vi "Valve automation test.vi"() -> ()   [LabVIEW 2016]
uses:
  <vilib>/Analysis/baseanly.llb/Mean (DBL).vi
  <vilib>/Analysis/NI_AALPro.lvlib
  <vilib>/Analysis/NI_AALBase.lvlib
  <vilib>/addons/control/pid/NI_PID_autopid.lvlib
panel:
  in  "PID gains":T1={"proportional gain (Kc)"=1.0, "integral time (Ti, min)"=0.01, "derivative time (Td, min)"=0.0} {"derivative time (Td, min)" format="%.3f"; "integral time (Ti, min)" format="%.3f"; "proportional gain (Kc)" format="%.3f"}
  out "PID gains out":T1={"proportional gain (Kc)"=1.0, "integral time (Ti, min)"=0.01, "derivative time (Td, min)"=0.0} {"derivative time (Td, min)" format="%.3f"; "integral time (Ti, min)" format="%.3f"; "proportional gain (Kc)" format="%.3f"}
  out "criterion":dbl
  out "output":dbl format="%.2f"
  out "new fill time":dbl
  out "abs error":dbl[unit]
  out "rate":dbl
  out "rel error":dbl
  in  "initial fill/vac tol":dbl
  in  "Samples to average":i32
  in  "Run":bool
  in  "Vacuum Cutoff":dbl[unit]
  in  "Fill Cutoff":dbl[unit]
  out "System Pressures":T2(graph)
  in  "Stop Button 2":bool
  in  "State":u16(ring) items=["Hold", "Vacuum", "Fill", "Vent"]
  out "Tube Inlet State":bool
  out "Mix Inlet State":bool
  out "Mix Outlet State":bool
  out "Tube Outlet State":bool
  out "Diluent State 2":bool caption="Diluent State"
  out "Vacuum State 2":bool caption="Vacuum State"
  out "Tube Pressure":dbl[unit]
  out "Manifold Pressure":dbl[unit]
  in  "Stop Button":bool
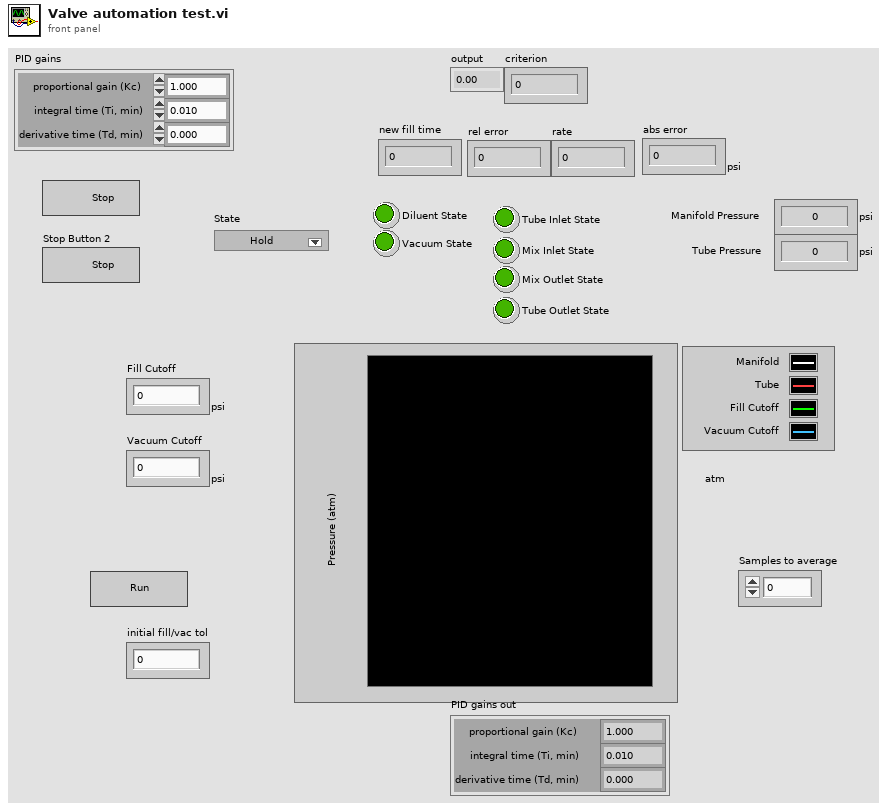
[diagram p1: front panel]
types:
  T1 = cluster{"proportional gain (Kc)":dbl, "integral time (Ti, min)":dbl, "derivative time (Td, min)":dbl}
  T2 = cluster{"Manifold Pressure":dbl[unit], "Tube Pressure":dbl[unit], "Fill Cutoff":dbl[unit], "Vacuum Cutoff":dbl[unit]}
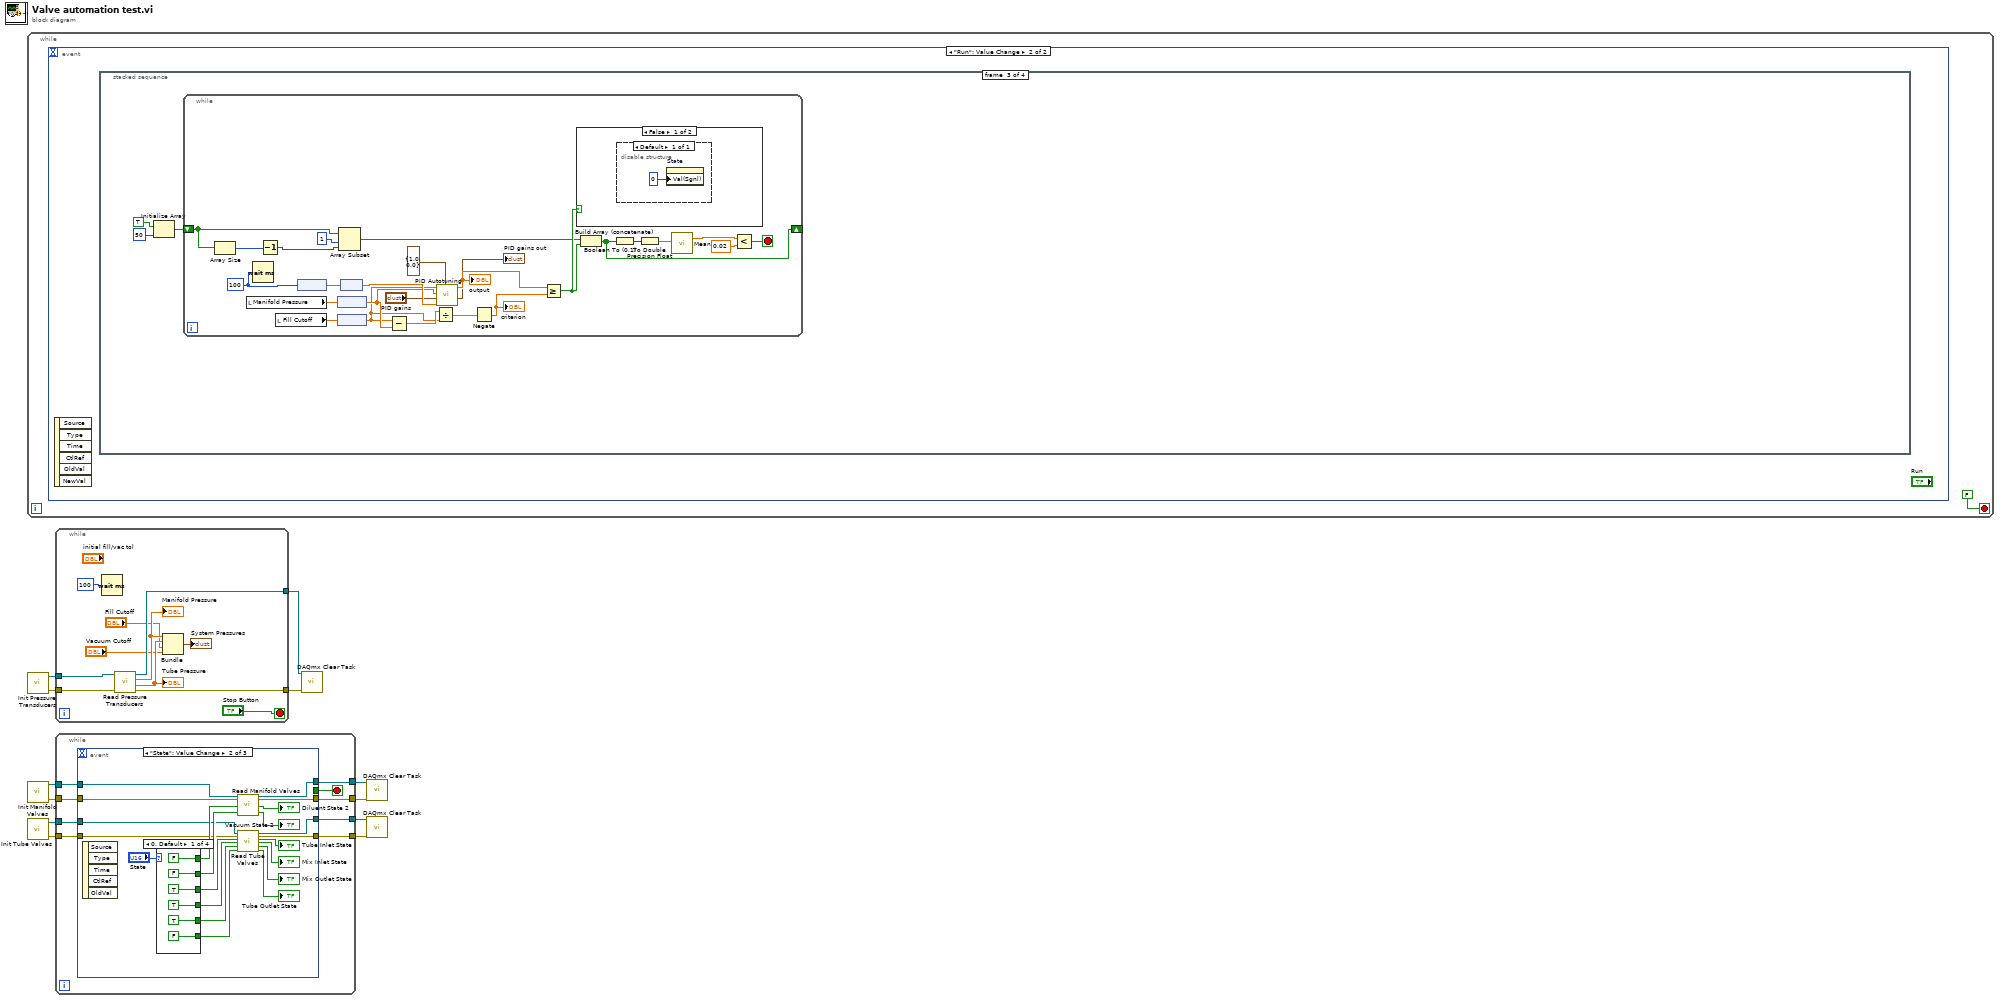
[diagram p0: block diagram]
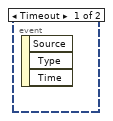
[diagram p2: hidden frame]
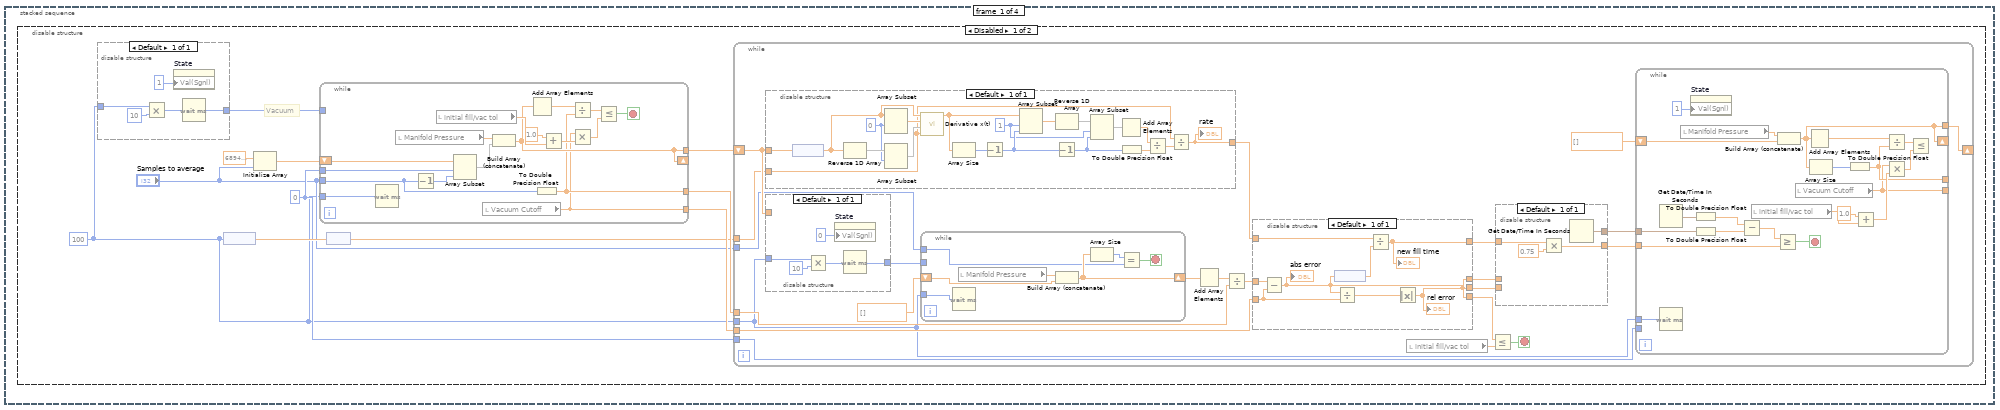
[diagram p3: hidden frame]
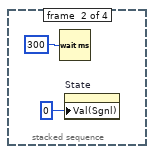
[diagram p5: hidden frame]
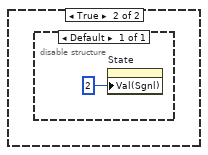
[diagram p6: hidden frame]
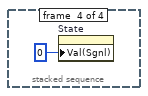
[diagram p7: hidden frame]
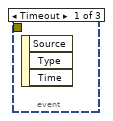
[diagram p8: hidden frame]
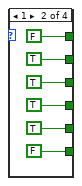
[diagram p9: hidden frame]
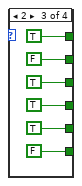
[diagram p10: hidden frame]
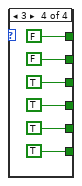
[diagram p11: hidden frame]
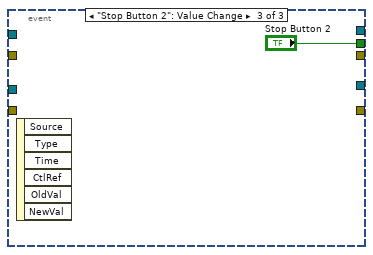
[diagram p12: hidden frame]
diagram:
  n1 = while {
    stop <- FALSE stop-if-true
    n2 = event shown="[1] \"Run\": Value Change" {
      selector: _ -> [_ _]
      dyn-events: _ -> [_ _]
      timeout: _ -> [_ _]
      event Timeout {
        n3 = event-data() -> ()  [unwired: 1 in, 3 out]
      }
      event "Run": Value Change {
        n4 = event-data() -> ()  [unwired: 1 in, 6 out]
        n5 = stacked-sequence {
          frame #0 {
            n6 = disable-structure shown="Disabled" {
              frame Disabled {
                w14 = u32 100 ("milliseconds to wait")
                w16 = 0 ("index")
                # "Vacuum"
                n7 = disable-structure shown="Default" {
                  disable-tunnel: w14 -> [w113]
                  disable-tunnel: [w112] -> w20
                  frame Enabled {
                    n8 = Multiply(x=w113, y=u32 10) -> (x*y=w115:u32)
                    n9 = property on="State" class="Ring (strict)"("Val(Sgnl)"=u16 1 ("Value (Signaling)")) -> ()  [unwired: 2 in, 2 out]
                    n10 = Wait (ms)(milliseconds to wait=w115) -> (millisecond timer value=w112:u32)
                  }
                }
                n11 = node(w14) -> (w19:dbl[unit])
                n12 = Initialize Array(dbl[unit] 6894757.88951578 ("element"), "Samples to average") -> (w24:dbl[unit][])
                n13 = while {
                  tunnel: w16 -> [w132]
                  tunnel: "Samples to average" -> [w127]
                  shift-right: [w119] -> _
                  shift-left: w24 -> [w130]
                  tunnel: w14 -> [w120]
                  tunnel: [w119] -> w18
                  tunnel: [w118] -> w22
                  tunnel: [w117] -> w21
                  tunnel: w20 -> [_]
                  stop <- w121 stop-if-true
                  n14 = Wait (ms)(milliseconds to wait=w120) -> ()  [unwired: 1 out]
                  n15 = local read "Manifold Pressure"() -> (w133:dbl[unit])
                  n16 = Decrement(x=w127) -> (x-1=w129:i32)
                  n17 = local read "initial fill/vac tol"() -> (w123:dbl)
                  n18 = Array Subset(array=w130, index=w132, length=w129) -> (w131:dbl[unit][])
                  n19 = local read "Vacuum Cutoff"() -> (w117:dbl[unit])
                  n20 = Build Array (concatenate)(w133, w131) -> (w119:dbl[unit][])
                  n21 = Add Array Elements(numeric array=w119) -> (sum=w128:dbl[unit])
                  n22 = To Double Precision Float(number=w127) -> (double precision float=w118:dbl)
                  n23 = Add(x=1.0, y=w123) -> (x+y=w124:dbl)
                  n24 = Divide(x=w128, y=w118) -> (x/y=w126:dbl[unit])
                  n25 = Multiply(x=w117, y=w124) -> (x*y=w125:dbl[unit])
                  n26 = Less Or Equal?(x=w126, y=w125) -> (x <= y?=w121:bool)
                }
                n27 = node(w19) -> (w17:dbl)
                n28 = while {
                  tunnel: w22 -> [w46]
                  tunnel: w21 -> [w45]
                  tunnel: w17 -> [w43]
                  tunnel: w16 -> [w35]
                  tunnel: "Samples to average" -> [w34]
                  tunnel: w14 -> [w33]
                  shift-right: [w28] -> _
                  shift-left: w18 -> [w44]
                  stop <- w25 stop-if-true
                  n29 = disable-structure shown="Default" {
                    disable-tunnel: w44 -> [w83]
                    disable-tunnel: w43 -> [w82]
                    disable-tunnel: [w81] -> w39
                    frame Enabled {
                      w93 = 1 ("index")
                      w84 = 0 ("index")
                      n30 = node(w83) -> (w86:dbl[])
                      n31 = Reverse 1D Array(array=w86) -> (reversed array=w85:dbl[])
                      n32 = Array Subset(array=w86, index=w84) -> (w87:dbl[])  [unwired: 1 in]
                      n33 = Array Subset(array=w85, index=w84) -> (w88:dbl[])  [unwired: 1 in]
                      n34 = call <vilib>:"Derivative x(t).vi"("dt"=w82, "Final Condition"=w88, "Initial Condition"=w87, "X"=w86) -> ("dX/dt"=w89:dbl[])  [unwired: 6 in, 1 out]
                      n35 = Array Size(array=w89) -> (size(s)=w90:i32)
                      n36 = Decrement(x=w90) -> (x-1=w94:i32)
                      n37 = Array Subset(array=w89, index=w93, length=w94) -> (w91:dbl[])
                      n38 = Reverse 1D Array(array=w91) -> (reversed array=w92:dbl[])
                      n39 = Decrement(x=w94) -> (x-1=w97:i32)
                      n40 = Array Subset(array=w92, index=w93, length=w97) -> (w95:dbl[])
                      n41 = Add Array Elements(numeric array=w95) -> (sum=w96:dbl)
                      n42 = To Double Precision Float(number=w97) -> (double precision float=w98:dbl)
                      n43 = Divide(x=w96, y=w98) -> (x/y=w99:dbl)
                      n44 = Divide(x=w82, y=w99) -> (x/y=w81:dbl)
                      "rate" <- w81
                    }
                  }
                  n45 = disable-structure shown="Default" {
                    disable-tunnel: w33 -> [w110]
                    disable-tunnel: [w107] -> w47
                    disable-tunnel: w44 -> [_]
                    frame Enabled {
                      n46 = Multiply(x=w110, y=u32 10) -> (x*y=w108:u32)
                      n47 = property on="State" class="Ring (strict)"("Val(Sgnl)"=u16 0 ("Value (Signaling)")) -> ()  [unwired: 2 in, 2 out]
                      n48 = Wait (ms)(milliseconds to wait=w108) -> (millisecond timer value=w107:u32)
                    }
                  }
                  n49 = while {
                    tunnel: w33 -> [w106]
                    tunnel: w47 -> [_]
                    shift-right: [w103] -> w32
                    shift-left: dbl[unit][] [] -> [w104]
                    tunnel: w34 -> [w101]
                    stop <- w100 stop-if-true
                    n50 = Wait (ms)(milliseconds to wait=w106) -> ()  [unwired: 1 out]
                    n51 = local read "Manifold Pressure"() -> (w105:dbl[unit])
                    n52 = Build Array (concatenate)(w105, w104) -> (w103:dbl[unit][])
                    n53 = Array Size(array=w103) -> (size(s)=w102:i32)
                    n54 = Equal?(x=w102, y=w101) -> (x = y?=w100:bool)
                  }
                  n55 = Add Array Elements(numeric array=w32) -> (sum=w41:dbl[unit])
                  n56 = Divide(x=w41, y=w46) -> (x/y=w40:dbl[unit])
                  n57 = disable-structure shown="Default" {
                    disable-tunnel: w45 -> [w80]
                    disable-tunnel: w40 -> [w79]
                    disable-tunnel: w39 -> [w78]
                    disable-tunnel: [w73] -> w38
                    disable-tunnel: [w76] -> w37
                    disable-tunnel: [w75] -> w36
                    disable-tunnel: [w73] -> w26
                    frame Enabled {
                      n58 = Subtract(x=w79, y=w80) -> (x-y=w76:dbl[unit])
                      "abs error" <- w76
                      n59 = node(w76) -> (w77:dbl)
                      n60 = Divide(x=w76, y=w80) -> (x/y=w74:dbl)
                      n61 = Divide(x=w78, y=w77) -> (x/y=w75:dbl)
                      "new fill time" <- w75
                      n62 = Absolute Value(x=w74) -> (abs(x)=w73:dbl)
                      "rel error" <- w73
                    }
                  }
                  n63 = local read "initial fill/vac tol"() -> (w27:dbl)
                  n64 = Less Or Equal?(x=w26, y=w27) -> (x <= y?=w25:bool)
                  n65 = disable-structure shown="Default" {
                    disable-tunnel: w38 -> [_]
                    disable-tunnel: w37 -> [_]
                    disable-tunnel: w36 -> [w71]
                    disable-tunnel: [w72] -> w31
                    disable-tunnel: [w70] -> w30
                    frame Enabled {
                      n66 = Multiply(x=w71, y=0.75) -> (x*y=w70:dbl)
                      n67 = Get Date/Time In Seconds() -> (seconds since 1Jan1904=w72:timestamp)
                    }
                  }
                  n68 = while {
                    tunnel: w35 -> [_]
                    shift-right: [w48] -> _
                    shift-left: dbl[unit][] [] -> [w50]
                    tunnel: w33 -> [w61]
                    tunnel: [w48] -> w28
                    tunnel: [w60] -> _
                    tunnel: [w59] -> _
                    tunnel: w31 -> [w53]
                    tunnel: w30 -> [w52]
                    stop <- w51 stop-if-true
                    n69 = Get Date/Time In Seconds() -> (seconds since 1Jan1904=w54:timestamp)
                    n70 = Wait (ms)(milliseconds to wait=w61) -> ()  [unwired: 1 out]
                    n71 = local read "Manifold Pressure"() -> (w68:dbl[unit])
                    n72 = property on="State" class="Ring (strict)"("Val(Sgnl)"=u16 1 ("Value (Signaling)")) -> ()  [unwired: 2 in, 2 out]
                    n73 = To Double Precision Float(number=w54) -> (double precision float=w56:dbl)
                    n74 = To Double Precision Float(number=w53) -> (double precision float=w55:dbl)
                    n75 = Subtract(x=w56, y=w55) -> (x-y=w57:dbl)
                    n76 = local read "initial fill/vac tol"() -> (w63:dbl)
                    n77 = Greater Or Equal?(x=w57, y=w52) -> (x >= y?=w51:bool)
                    n78 = Build Array (concatenate)(w68, w50) -> (w48:dbl[unit][])
                    n79 = local read "Vacuum Cutoff"() -> (w59:dbl[unit])
                    n80 = Add Array Elements(numeric array=w48) -> (sum=w67:dbl[unit])
                    n81 = Array Size(array=w48) -> (size(s)=w49:i32)
                    n82 = To Double Precision Float(number=w49) -> (double precision float=w60:dbl)
                    n83 = Add(x=1.0, y=w63) -> (x+y=w64:dbl)
                    n84 = Divide(x=w67, y=w60) -> (x/y=w66:dbl[unit])
                    n85 = Multiply(x=w59, y=w64) -> (x*y=w65:dbl[unit])
                    n86 = Less Or Equal?(x=w66, y=w65) -> ()  [unwired: 1 out]
                  }
                }
              }
              frame Enabled {
              }
            }
          }
          frame #1 {
            n87 = Wait (ms)(milliseconds to wait=u32 300) -> ()  [unwired: 1 out]
            n88 = property on="State" class="Ring (strict)"("Val(Sgnl)"=u16 0 ("Value (Signaling)")) -> ()  [unwired: 2 in, 2 out]
          }
          frame #2 {
            n89 = Initialize Array(TRUE, 50 ("dimension size")) -> (w138:bool[])
            n90 = while {
              shift-right: [w155] -> _
              shift-left: w138 -> [w150]
              stop <- w143 stop-if-true
              w162 = u32 100 ("milliseconds to wait")
              n91 = Array Size(array=w150) -> (size(s)=w149:i32)
              n92 = local read "Manifold Pressure"() -> (w158:dbl[unit])
              n93 = Wait (ms)(milliseconds to wait=w162) -> ()  [unwired: 1 out]
              n94 = Decrement(x=w149) -> (x-1=w148:i32)
              n95 = local read "Fill Cutoff"() -> (w159:dbl[unit])
              n96 = node(w162) -> (w164:dbl[unit])
              n97 = node(w158) -> (w147:dbl)
              n98 = node(w159) -> (w140:dbl)
              n99 = Array Subset(array=w150, index=1, length=w148) -> (w156:bool[])
              n100 = node(w164) -> (w163:dbl)
              n101 = Subtract(x=w140, y=w147) -> (x-y=w142:dbl)
              n102 = Divide(x=w142, y=w140) -> (x/y=w141:dbl)
              n103 = call <vilib>:"PID Autotuning.vi"("output range"=cluster{"output high":dbl, "output low":dbl} {"output high"=1.0, "output low"=0.0}, "dt (s)"=w163, "PID gains"="PID gains", "process variable"=w147, "setpoint"=w140) -> ("PID gains out"=→"PID gains out":T1, "output"=w146:dbl)  [unwired: 3 in, 2 out]
              "output" <- w146
              n104 = Negate(x=w141) -> (-x=w145:dbl)
              "criterion" <- w145
              n105 = Greater Or Equal?(x=w146, y=w145) -> (x >= y?=w157:bool)
              n106 = case shown="False" w157 {
                frame False {
                  n107 = disable-structure shown="Default" {
                    frame Enabled {
                      n108 = property on="State" class="Ring (strict)"("Val(Sgnl)"=u16 0 ("Value (Signaling)")) -> ()  [unwired: 2 in, 2 out]
                    }
                  }
                }
                frame True {
                  n109 = disable-structure shown="Default" {
                    frame Enabled {
                      n110 = property on="State" class="Ring (strict)"("Val(Sgnl)"=u16 2 ("Value (Signaling)")) -> ()  [unwired: 2 in, 2 out]
                    }
                  }
                }
              }
              n111 = Build Array (concatenate)(w156, w157) -> (w155:bool[])
              n112 = Boolean To (0,1)(Boolean=w155) -> (0, 1=w154:i16[])
              n113 = To Double Precision Float(number=w154) -> (double precision float=w153:dbl[])
              n114 = call-poly <vilib>:"Mean.vi"("X"=w153) -> ("mean"=w152:dbl)  [unwired: 1 out]
              n115 = Less?(x=w152, y=0.02) -> (x < y?=w143:bool)
            }
          }
          frame #3 {
            n116 = property on="State" class="Ring (strict)"("Val(Sgnl)"=u16 0 ("Value (Signaling)")) -> ()  [unwired: 2 in, 2 out]
          }
        }
      }
    }
  }
  n117 = call "Init Pressure Transducers.vi"() -> ("Error Out"=w11:errorcluster, "task out"=w12:refnum<k21>)  [unwired: 1 in]
  n118 = call "Init Manifold Valves.vi"() -> ("Error Out"=w7:errorcluster, "task out"=w8:refnum<k21>)  [unwired: 1 in]
  n119 = call "Init Tube Valves.vi"() -> ("Error Out"=w5:errorcluster, "task out"=w6:refnum<k21>)  [unwired: 1 in]
  n120 = while {
    tunnel: w12 -> [w178]
    tunnel: w11 -> [w177]
    tunnel: [w175] -> w10
    tunnel: [w174] -> w9
    stop <- "Stop Button" stop-if-true
    n121 = Wait (ms)(milliseconds to wait=u32 100) -> ()  [unwired: 1 out]
    n122 = call "Read Pressure Transducers.vi"("Error In"=w177, "task in"=w178) -> ("Error Out"=w174:errorcluster, "Tube Pressure"=w171:dbl[unit], "Manifold Pressure"=w172:dbl[unit], "task out"=w175:refnum<k21>)  [unwired: 5 in, 1 out]
    "Manifold Pressure" <- w172
    "Tube Pressure" <- w171
    n123 = Bundle("Manifold Pressure"=w172, "Tube Pressure"=w171, "Fill Cutoff"="Fill Cutoff", "Vacuum Cutoff"="Vacuum Cutoff") -> (→"System Pressures":T2)  [unwired: 1 in]
  }
  n124 = while {
    tunnel: w8 -> [w187]
    tunnel: w7 -> [w186]
    tunnel: w6 -> [w185]
    tunnel: w5 -> [w184]
    tunnel: [w183] -> w4
    tunnel: [w182] -> w3
    tunnel: [w181] -> w2
    tunnel: [w180] -> w1
    stop <- w179 stop-if-true
    n125 = event shown="[1] \"State\": Value Change" {
      selector: _ -> [_ _ _]
      dyn-events: _ -> [_ _ _]
      timeout: _ -> [_ _ _]
      tunnel: [_ w208 _] -> w183
      tunnel: [_ w207 _] -> w182
      tunnel: [_ w206 _] -> w181
      tunnel: [_ w205 _] -> w180
      tunnel: w187 -> [_ w191 _]
      tunnel: w186 -> [_ w190 _]
      tunnel: w185 -> [_ w189 _]
      tunnel: w184 -> [_ w188 _]
      tunnel: [_ _ "Stop Button 2"] -> w179
      event Timeout {
        n126 = event-data() -> ()  [unwired: 1 in, 3 out]
      }
      event "State": Value Change {
        n127 = event-data() -> ()  [unwired: 1 in, 5 out]
        n128 = case shown="0, Default" "State" {
          tunnel: [TRUE TRUE TRUE TRUE] -> w203
          tunnel: [TRUE TRUE TRUE TRUE] -> w202
          tunnel: [TRUE TRUE TRUE TRUE] -> w201
          tunnel: [FALSE FALSE FALSE TRUE] -> w200
          tunnel: [FALSE FALSE TRUE FALSE] -> w199
          tunnel: [FALSE TRUE FALSE FALSE] -> w198
          frame 0, Default {
          }
          frame 1 {
          }
          frame 2 {
          }
          frame 3 {
          }
        }
        n129 = call "Read Manifold Valves.vi"("Task In"=w191, "Error In"=w190, "Diluent"=w199, "Vacuum"=w198) -> ("Task Out"=w208:refnum<k21>, "Error Out"=w207:errorcluster, "Diluent State"=→"Diluent State 2":bool, "Vacuum State"=→"Vacuum State 2":bool)  [unwired: 16 in, 4 out]
        n130 = call "Read Tube Valves.vi"("task in"=w189, "Error In"=w188, "Tube Inlet"=w203, "Mix Inlet"=w202, "Mix Outlet"=w201, "Tube Outlet"=w200) -> ("task out"=w206:refnum<k21>, "Error Out"=w205:errorcluster, "Tube Inlet State"=→"Tube Inlet State":bool, "Mix Inlet State"=→"Mix Inlet State":bool, "Mix Outlet State"=→"Mix Outlet State":bool, "Tube Outlet State"=→"Tube Outlet State":bool)  [unwired: 8 in]
      }
      event "Stop Button 2": Value Change {
        n131 = event-data() -> ()  [unwired: 1 in, 6 out]
      }
    }
  }
  n132 = call <vilib>:"DAQmx Clear Task.vi"("task in"=w10, "error in"=w9) -> ()  [unwired: 13 in, 1 out]
  n133 = call <vilib>:"DAQmx Clear Task.vi"("task in"=w4, "error in"=w3) -> ()  [unwired: 13 in, 1 out]
  n134 = call <vilib>:"DAQmx Clear Task.vi"("task in"=w2, "error in"=w1) -> ()  [unwired: 13 in, 1 out]
